vi "Write Digital Outputs.vi"(8 "error in (no error)":errorcluster, 9 "Device Number":string, 10 "Digital Outputs":bool[](array[boolean]), 11 "VISA resource name":refnum<visa-resource-name>) -> (0 "error out":errorcluster, 3 "VISA resource name out":refnum<visa-resource-name>)   [LabVIEW 2013, in "Zaber A Series.lvlib"]
doc: "Writes to the digital output pins on a Zaber controller device such as the A-MCB or X-MCB series devices. Input is an array of booleans that must have the same number of elements as there are digital output pins on the device - use the Get I/O Pin Counts VI to determine this.\n \nThis VI requires that the Initialize VI has been called with the same serial port."
uses:
  Zaber A Series.lvlib
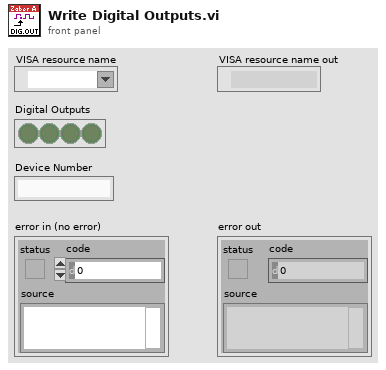
[diagram p1: front panel]
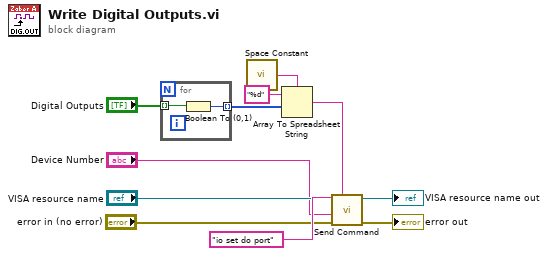
[diagram p0: block diagram]
diagram:
  n1 = for {
    tunnel: "Digital Outputs" -> [w13] mode=indexing
    tunnel: [w12] -> w7 mode=indexing
    n2 = Boolean To (0,1)(Boolean=w13) -> (0, 1=w12:i16)
  }
  n3 = call <vilib>:"Space Constant.vi"() -> ("String"=w5:string)
  n4 = Array To Spreadsheet String(delimiter (Tab)=w5, array=w7, 3:"%d" ("format string")) -> (spreadsheet string=w4:string)
  n5 = call "Send Command.vi"("Data"=w4, "error in (no error)"="error in (no error)", "Device and Axis"="Device Number", "Command"="io set do port" ("Complete Command List"), "VISA resource name"="VISA resource name") -> ("error out"=→"error out":errorcluster, "VISA resource name out"=→"VISA resource name out":refnum<visa-resource-name>)  [unwired: 1 in, 4 out]
